vi "Test MQTT-2.3.1-6.vi"(8 "error in (no error)":errorcluster) -> (0 "error out":errorcluster)   [LabVIEW 2013]
uses:
  source/Control Packets/ControlPacket/QualityOfService -- enum.ctl
  <vilib>/addons/_JKI Toolkits/Caraya/classes/Test/Test.lvclass
  <vilib>/addons/_JKI Toolkits/Caraya/classes/Assert/Assert.lvclass
  source/Client/Client.lvclass
  source/MQTT_Base/MQTT_Base.lvclass
  source/Control Packets/ControlPacket/ControlPacket.lvclass
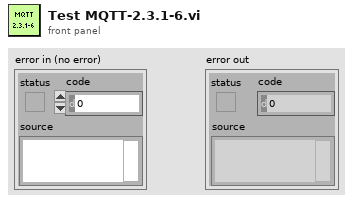
[diagram p1: front panel]
types:
  T1 = typedef "ControlPacket.lvclass/QualityOfService -- enum.ctl" = enum16{"0 (At Most Once)", "1 (At Least Once)", "2 (Exactly Once)"}
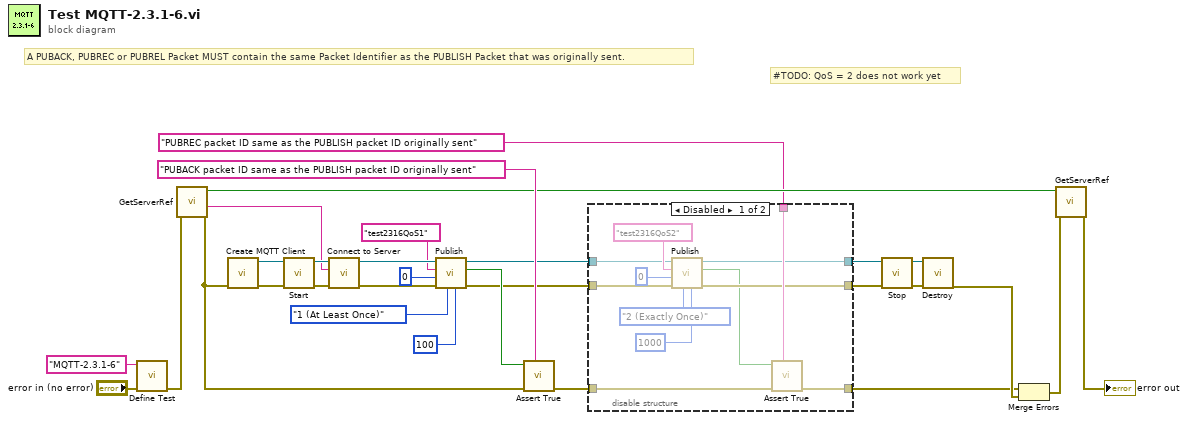
[diagram p0: block diagram]
diagram:
  # "#TODO: QoS = 2 does not work yet"
  # "A PUBACK, PUBREC or PUBREL Packet MUST contain the same Packet Identifier as the PUBLISH Packet that was originally sent."
  n1 = call <vilib>:"Define Test.vi"("error in (no error)"="error in (no error)", "Label (VI Title)"="MQTT-2.3.1-6") -> ("error out"=w27:errorcluster)  [unwired: 9 in]
  n2 = call "GetServerRef.vi"("error in"=w27) -> ("error out"=w19:errorcluster, "Server address"=w15:string, "Created"=w26:bool)  [unwired: 7 in, 1 out]
  n3 = call "Create MQTT Client.vi"("error in (no error)"=w19) -> ("error out"=w20:errorcluster, "Client out"=w21:refnum<class "Client.lvclass">)  [unwired: 9 in]
  n4 = call "Start.vi"("error in (no error)"=w20, "MQTT_Base in"=w21) -> ("error out"=w23:errorcluster, "MQTT_Base out"=w24:refnum<class "Client.lvclass">)  [unwired: 7 in, 1 out]
  n5 = call "Connect to Server.vi"("error in (no error)"=w23, "address (localhost)"=w15, "Client in"=w24) -> ("error out"=w13:errorcluster, "Client out"=w14:refnum<class "Client.lvclass">)  [unwired: 5 in, 2 out]
  n6 = call "Publish.vi"("timeout (1000ms)"=100, "QoS"=QualityOfService_--_enum."1 (At Least Once)", "error in (no error)"=w13, "Payload"=0, "Topic Name (empty: Payload name)"="test2316QoS1", "Client in"=w14) -> ("error out"=w4:errorcluster, "Published"=w9:bool, "Client out"=w5:refnum<class "Client.lvclass">)  [unwired: 3 in]
  n7 = call <vilib>:"Assert True.vi"("Label"="PUBACK packet ID same as the PUBLISH packet ID originally sent", "error in (no error)"=w19, "True?"=w9) -> ("error out"=w8:errorcluster)  [unwired: 8 in]
  n8 = disable-structure shown="Disabled" {
    disable-tunnel: w8 -> [w42 w43]
    disable-tunnel: [w41 w43] -> w7
    disable-tunnel: "PUBREC packet ID same as the PUBLISH packet ID originally sent" ("Label") -> [w40 _]
    disable-tunnel: w5 -> [w36 w45]
    disable-tunnel: w4 -> [w35 w44]
    disable-tunnel: [w34 w45] -> w3
    disable-tunnel: [w33 w44] -> w2
    frame Disabled {
      n9 = call "Publish.vi"("timeout (1000ms)"=1000, "QoS"=QualityOfService_--_enum."2 (Exactly Once)", "error in (no error)"=w35, "Payload"=0, "Topic Name (empty: Payload name)"="test2316QoS2", "Client in"=w36) -> ("error out"=w33:errorcluster, "Published"=w32:bool, "Client out"=w34:refnum<class "Client.lvclass">)  [unwired: 3 in]
      n10 = call <vilib>:"Assert True.vi"("Label"=w40, "error in (no error)"=w42, "True?"=w32) -> ("error out"=w41:errorcluster)  [unwired: 8 in]
    }
    frame Enabled {
    }
  }
  n11 = call "Stop.vi"("error in (no error)"=w2, "MQTT_Base in"=w3) -> ("error out"=w16:errorcluster, "MQTT_Base out"=w22:refnum<class "Client.lvclass">)  [unwired: 7 in, 1 out]
  n12 = call "Destroy.vi"("error in (no error)"=w16, "MQTT_Base in"=w22) -> ("error out"=w18:errorcluster)  [unwired: 8 in, 1 out]
  n13 = Merge Errors(w7, w18) -> (w17:errorcluster)
  n14 = call "GetServerRef.vi"("error in"=w17, "Destroy (F)"=w26) -> ("error out"=→"error out":errorcluster)  [unwired: 6 in, 3 out]
